vi "test3subci.vi"(8 "error in (no error)":errorcluster, 10 "fmt":T1(ring), 11 "index":i32) -> (0 "error out":errorcluster, 3 "Destination":u16[](array[numeric]))   [LabVIEW 2012]
uses:
  Public/lib/freenect_sync.dll
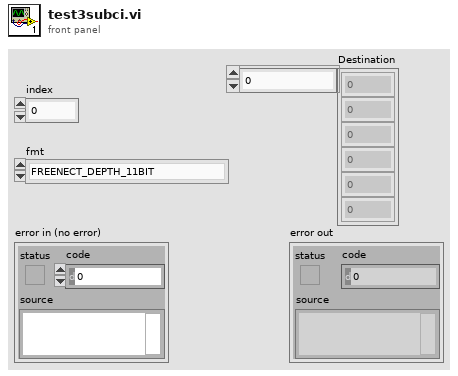
[diagram p1: front panel]
types:
  T1 = enum16{"FREENECT_DEPTH_11BIT", "FREENECT_DEPTH_10BIT", "FREENECT_DEPTH_11BIT_PACKED", "FREENECT_DEPTH_10BIT_PACKED"}
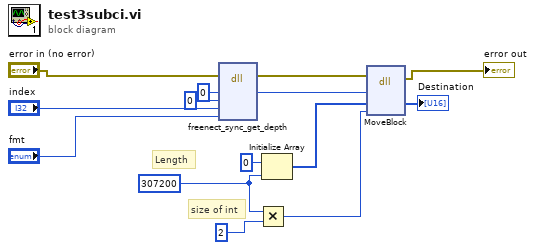
[diagram p0: block diagram]
diagram:
  w7 = 307200 ("dimension size")
  # "size of int"
  # "Length"
  n1 = dll-call lib="C:/Program Files/National Instruments/LabVIEW 2011/vi.lib/LabVIEW Hacker/LVH-Interface-for-Kinect/Public/lib/freenect_sync.dll" fn="freenect_sync_get_depth"(error in="error in (no error)", "ptr"=i64 0, "timestamp"=u32 0, "index"="index", "fmt"="fmt") -> (error out=w10:errorcluster, "ptr"=w3:i64)  [unwired: 3 in, 4 out]
  n2 = Multiply(x=w7, y=2) -> (x*y=w5:i32)
  n3 = Initialize Array(u16 0 ("element"), w7) -> (w8:u16[])
  n4 = dll-call lib="LabVIEW" fn="MoveBlock"(error in=w10, "Address (Pointer)"=w3, "Destination"=w8, "Size"=w5) -> (error out=→"error out":errorcluster, "Destination"=→"Destination":u16[])  [unwired: 4 in, 2 out]
